vi "gj.vi"() -> ()   [LabVIEW 2014]
panel:
  out "Array 2":dbl[][](array[numeric])
  in  "Array":dbl[][](array[numeric])
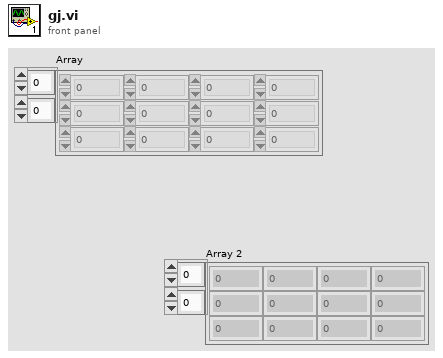
[diagram p1: front panel]
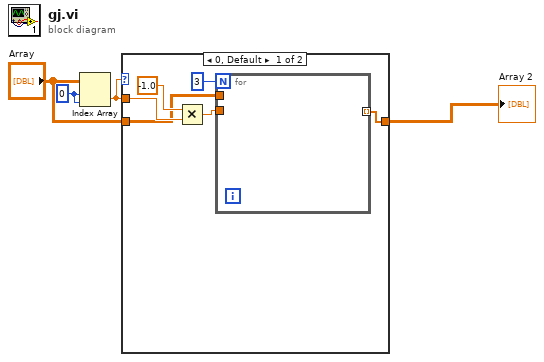
[diagram p0: block diagram]
diagram:
  w4 = 0 ("index (row)")
  n1 = Index Array(array="Array", index (row)=w4, index (col)=w4) -> (element=w3:dbl)
  n2 = case shown="0, Default" w3 {
    tunnel: w3 -> [w10 _]
    tunnel: "Array" -> [w7 w12]
    tunnel: [w5 w12] -> w1
    frame 0, Default {
      n3 = Multiply(x=-1.0, y=w10) -> (x*y=w6:dbl)
      n4 = for {
        N: 3 -> [_]
        tunnel: w7 -> [_]
        tunnel: w6 -> [_]
        tunnel: [w11] -> w5 mode=indexing
      }
    }
    frame 1 {
    }
  }
  "Array 2" <- w1
